vi "Step Get By Sequence and Index.vi"(8 "error in (no error)":errorcluster, 9 "iIndex":i32, 10 "sxSequenceID":string, 11 "Connection Refnum":T2) -> (0 "error out":errorcluster, 2 "Step Record":T1, 3 "Connection Refnum":T2, 4 "Data Present":bool)   [LabVIEW 2011]
uses:
  Summitek EXT/ODBC/SQL Controls/Connection Refnum.ctl
  Step Record.ctl
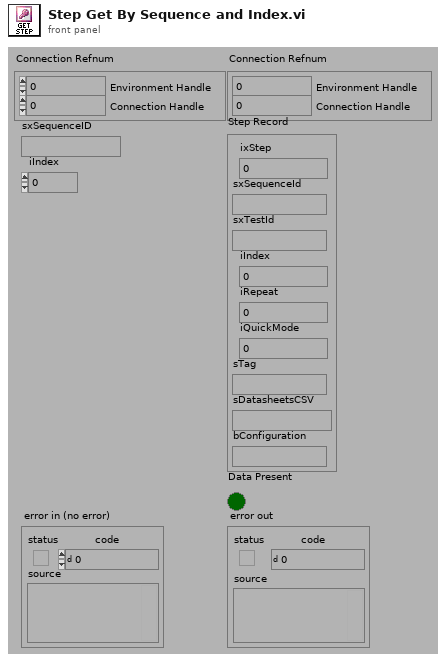
[diagram p1: front panel]
types:
  T1 = typedef "Step Record.ctl" = cluster{"ixStep":i32, "sxSequenceId":string, "sxTestId":string, "iIndex":i32, "iRepeat":i32, "iQuickMode":i32, "sTag":string, "sDatasheetsCSV":string, "bConfiguration":string}
  T2 = typedef "Connection Refnum.ctl" = cluster{"Environment Handle":i32, "Connection Handle":i32}
  T3 = typedef "Statement Refnum.ctl" = cluster{"Statement Handle":i32, "Parameter Number":u16}
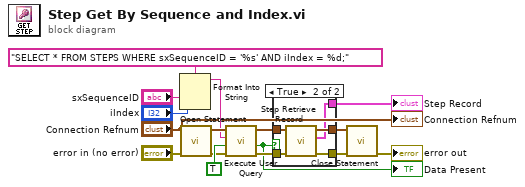
[diagram p0: block diagram]
diagram:
  n1 = Format Into String(format string="SELECT * FROM STEPS WHERE sxSequenceID = '%s' AND iIndex = %d;" ("User Query"), "sxSequenceID", "iIndex") -> (resulting string=w9:string)  [unwired: 2 in, 1 out]
  n2 = call "Open Statement.vi"("error in (no error)"="error in (no error)", "Connection Refnum"="Connection Refnum") -> ("error out"=w10:errorcluster, "Statement Refnum"=w11:T3)  [unwired: 4 out]
  n3 = call "Execute User Query.vi"("error in (no error)"=w10, "Return Data? (f)"=TRUE, "User Query"=w9, "Statement Refnum"=w11) -> ("error out"=w16:errorcluster, "Data Present?"=w8:bool, "Statement Refnum"=w15:T3)  [unwired: 1 out]
  "Data Present" <- w8
  n4 = case shown="True" w8 {
    tunnel: w16 -> [w17 w22]
    tunnel: w15 -> [w18 w23]
    tunnel: [w17 w20] -> w12
    tunnel: [w18 w21] -> w13
    tunnel: [_ w19] -> w5
    frame False {
    }
    frame True {
      n5 = call "Step Retrieve Record.vi"("error in (no error)"=w22, "Statement Refnum"=w23) -> ("error out"=w20:errorcluster, "Step"=w19:T1, "Statement Refnum"=w21:T3)  [unwired: 7 out]
    }
  }
  "Step Record" <- w5
  n6 = call "Close Statement.vi"("error in (no error)"=w12, "Statement Refnum"=w13) -> ("error out"=→"error out":errorcluster)  [unwired: 5 out]
  "Connection Refnum" <- "Connection Refnum"
